vi "Write Rects.vi"(8 "error in (no error)":errorcluster, 10 "Rects":T1[](array[typedef]), 11 "ParseSVG in":refnum<class "ParseSVG.lvclass">) -> (0 "error out":errorcluster, 3 "ParseSVG out":refnum<class "ParseSVG.lvclass">)   [LabVIEW 2019, in "ParseSVG.lvclass"]
uses:
  ParseSVG.lvclass
  Rect.ctl
  ParseSVG.lvclass/ParseSVG.ctl
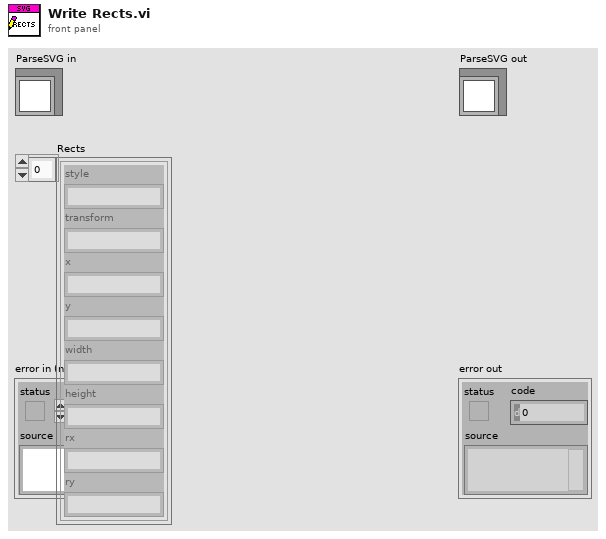
[diagram p1: front panel]
types:
  T1 = typedef "ParseSVG.lvclass/Rect.ctl" = cluster{"style":string, "transform":string, "x":string, "y":string, "width":string, "height":string, "rx":string, "ry":string}
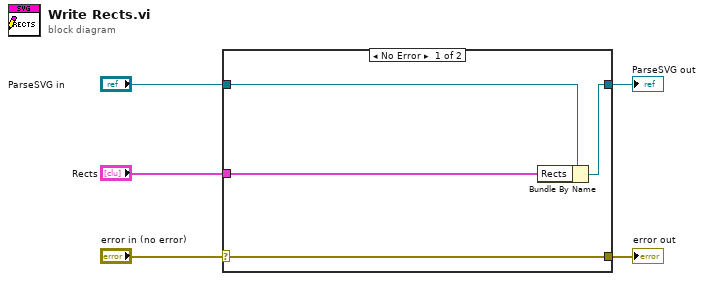
[diagram p0: block diagram]
diagram:
  n1 = case shown="No Error" "error in (no error)" {
    selector: "error in (no error)" -> [w9 w10]
    tunnel: [w9 w10] -> w4
    tunnel: [w7 w11] -> w2
    tunnel: "ParseSVG in" -> [w8 w11]
    tunnel: "Rects" -> [w6 _]
    frame No Error {
      n2 = Bundle By Name(cluster=w8, "Rects"=w6) -> (w7:refnum<class "ParseSVG.lvclass">)
    }
    frame Error {
    }
  }
  "error out" <- w4
  "ParseSVG out" <- w2
